vi "Agebraic Berechnung.vi"(8 "X Values":sgl[](array[numeric]) caption="X-Werte" format="%0.2f", 9 "Variables":string[](array[string]) caption="Variablen", 11 "formula":string caption="Formel") -> (0 "error out":errorcluster caption="Fehler (Ausgang)", 3 "y value":sgl)   [LabVIEW 2020, in "FT-IR.lvlib" / "Algebraic Modul.lvlib"]
uses:
  Algebraic Modul.lvlib
  <vilib>/gmath/NI_Gmath.lvlib
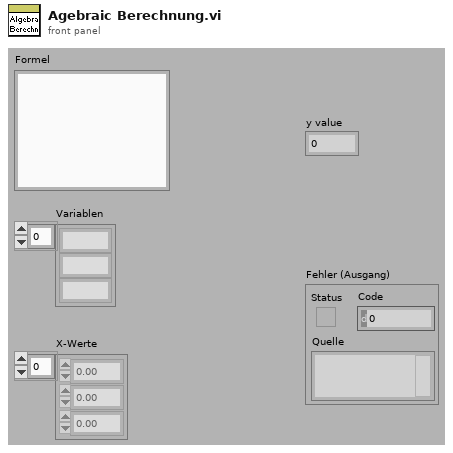
[diagram p1: front panel]
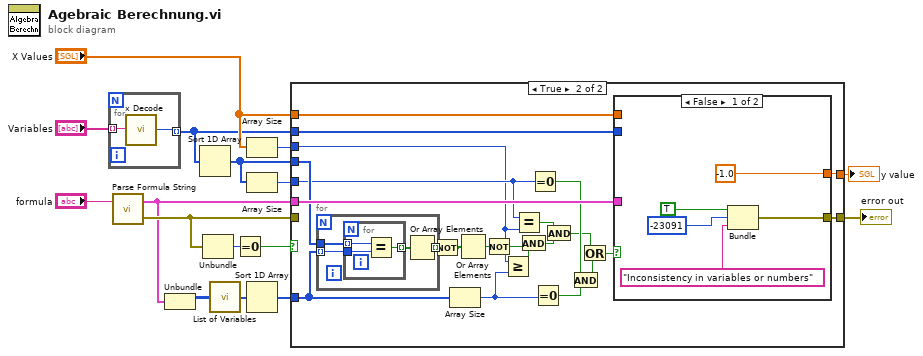
[diagram p0: block diagram]
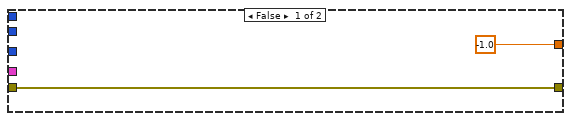
[diagram p2: hidden frame]
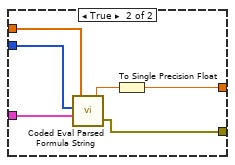
[diagram p3: hidden frame]
diagram:
  n1 = for {
    tunnel: "Variables" -> [w18] mode=indexing
    tunnel: [w17] -> w4 mode=indexing
    n2 = call <vilib>:"x Decode.vi"("x string"=w18) -> ("number"=w17:i32)  [unwired: 1 in, 1 out]
  }
  n3 = call <vilib>:"Parse Formula String.vi"("formula"="formula") -> ("error out"=w7:errorcluster, "Parsed Formula"=w3:cluster{"Table":i32[][], "Y Values":dbl[]})  [unwired: 1 in]
  n4 = Unbundle(w3) -> ("Table"=w12:i32[][])  [unwired: 1 out]
  n5 = Sort 1D Array(array=w4) -> (sorted array=w9:i32[])
  n6 = Unbundle(w7) -> ("code"=w8:i32)  [unwired: 2 out]
  n7 = call <vilib>:"List of Variables.vi"("Table"=w12) -> ("List of variables"=w5:i32[])
  n8 = Equal To 0?(x=w8) -> (x = 0?=w1:bool)
  n9 = Array Size(array="X Values") -> (size(s)=w6:i32)
  n10 = Array Size(array=w9) -> (size(s)=w10:i32)
  n11 = Sort 1D Array(array=w5) -> (sorted array=w11:i32[])
  n12 = case shown="True" w1 {
    tunnel: [sgl -1.0 w42] -> w16
    tunnel: w7 -> [w20 _]
    tunnel: w3 -> [_ w41]
    tunnel: "X Values" -> [_ w38]
    tunnel: w4 -> [_ w40]
    tunnel: w9 -> [_ w33]
    tunnel: w11 -> [_ w34]
    tunnel: w6 -> [_ w23]
    tunnel: [w20 w22] -> w2
    tunnel: w10 -> [_ w31]
    frame False {
    }
    frame True {
      n13 = for {
        tunnel: w34 -> [w46] mode=indexing
        tunnel: w33 -> [w45]
        tunnel: [w43] -> w32 mode=indexing
        n14 = for {
          tunnel: w46 -> [w49]
          tunnel: w45 -> [w48] mode=indexing
          tunnel: [w47] -> w44 mode=indexing
          n15 = Equal?(x=w48, y=w49) -> (x = y?=w47:bool)
        }
        n16 = Or Array Elements(Boolean array=w44) -> (logical OR=w43:bool)
      }
      n17 = Not(x=w32) -> (.not. x?=w24:bool[])
      n18 = Array Size(array=w34) -> (size(s)=w37:i32)
      n19 = Or Array Elements(Boolean array=w24) -> (logical OR=w25:bool)
      n20 = Not(x=w25) -> (.not. x?=w21:bool)
      n21 = Greater Or Equal?(x=w23, y=w37) -> (x >= y?=w39:bool)
      n22 = Equal?(x=w31, y=w23) -> (x = y?=w36:bool)
      n23 = And(x=w21, y=w39) -> (x .and. y?=w35:bool)
      n24 = Equal To 0?(x=w31) -> (x = 0?=w30:bool)
      n25 = Equal To 0?(x=w37) -> (x = 0?=w29:bool)
      n26 = And(x=w36, y=w35) -> (x .and. y?=w28:bool)
      n27 = And(x=w30, y=w29) -> (x .and. y?=w27:bool)
      n28 = Or(x=w28, y=w27) -> (x .or. y?=w26:bool)
      n29 = case shown="False" w26 {
        tunnel: w38 -> [_ w60]
        tunnel: [sgl -1.0 w57] -> w42
        tunnel: w41 -> [_ w56]
        tunnel: w40 -> [_ w59]
        tunnel: [w50 w55] -> w22
        frame False {
          n30 = Bundle(TRUE, -23091, "Inconsistency in variables or numbers") -> (w50:errorcluster)  [unwired: 1 in]
        }
        frame True {
          n31 = call <vilib>:"Coded Eval Parsed Formula String.vi"("Parsed Formula"=w56, "Variables"=w59, "X Values"=w60) -> ("error out"=w55:errorcluster, "y value"=w58:dbl)  [unwired: 1 in]
          n32 = To Single Precision Float(number=w58) -> (single precision float=w57:sgl)
        }
      }
    }
  }
  "error out" <- w2
  "y value" <- w16
